vi "Draw Trajectory.vi"(9 "dt":dbl, 10 "Array":dbl[](array[numeric]), 11 "# Points":i32) -> (3 "Cluster":cluster{dbl[], dbl[]})   [LabVIEW 2020]
uses:
  <vilib>/Analysis/coordinate.llb/2D Cartesian Coordinate Rotation (Scalar).vi
  <vilib>/Analysis/NI_AALPro.lvlib
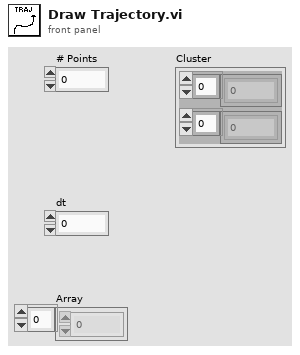
[diagram p1: front panel]
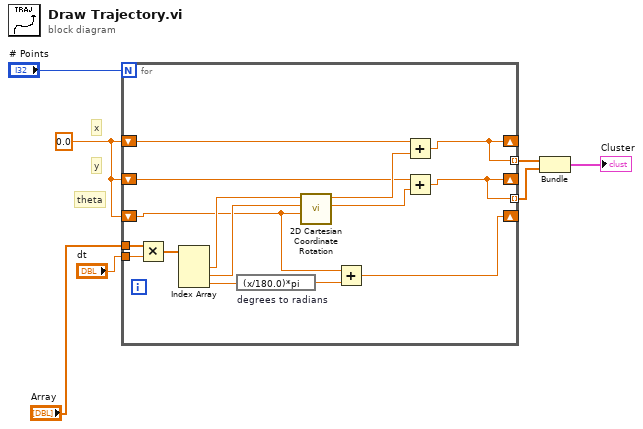
[diagram p0: block diagram]
diagram:
  w3 = 0.0 ("dt")
  # "theta"
  # "y"
  # "x"
  n1 = for {
    N: "# Points" -> [_]
    shift-right: [w9] -> _
    shift-left: w3 -> [w16]
    shift-right: [w8] -> _
    shift-left: w3 -> [w14]
    shift-right: [w10] -> _
    shift-left: w3 -> [w11]
    tunnel: "Array" -> [w21]
    tunnel: "dt" -> [w19]
    tunnel: [w9] -> w5 mode=indexing
    tunnel: [w8] -> w6 mode=indexing
    n2 = Multiply(x=w21, y=w19) -> (x*y=w20:dbl[])
    n3 = Index Array(array=w20) -> (element #1=w18:dbl, element #2=w17:dbl, element #3=w22:dbl)  [unwired: 3 in]
    n4 = expression code="(x/180.0)*pi" "degrees to radians"(w22) -> (w12:dbl)
    n5 = call-poly <vilib>:"2D Cartesian Coordinate Rotation.vi"("theta"=w11, "y"=w17, "x"=w18) -> ("y out"=w13:dbl, "x out"=w15:dbl)  [unwired: 6 in, 1 out]
    n6 = Add(x=w11, y=w12) -> (x+y=w10:dbl)
    n7 = Add(x=w16, y=w15) -> (x+y=w9:dbl)
    n8 = Add(x=w14, y=w13) -> (x+y=w8:dbl)
  }
  n9 = Bundle(w5, w6) -> (→"Cluster":cluster{dbl[], dbl[]})  [unwired: 1 in]
